vi "set_size.vi"(8 "error in (no error)":errorcluster, 9 "y":i32, 10 "x":i32, 11 "Image in":refnum<class "Image.lvclass">) -> (0 "error out":errorcluster, 3 "Image out":refnum<class "Image.lvclass">)   [LabVIEW 2010, in "Image.lvclass"]
uses:
  Image.lvclass
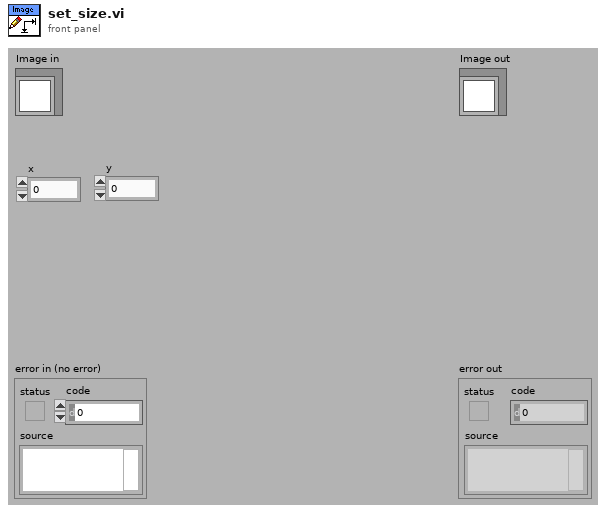
[diagram p1: front panel]
types:
  T1 = typedef "IMAQ Image.ctl" = refnum<image>
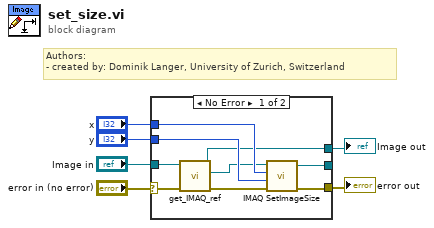
[diagram p0: block diagram]
diagram:
  # "Authors: \n- created by: Dominik Langer, University of Zurich, Switzerland"
  n1 = case shown="No Error" "error in (no error)" {
    selector: "error in (no error)" -> [w14 w17]
    tunnel: [w15 w17] -> w5
    tunnel: [w8 w16] -> w3
    tunnel: "Image in" -> [w12 w16]
    tunnel: "x" -> [w11 _]
    tunnel: "y" -> [w10 _]
    tunnel: [w7 _] -> _
    frame No Error {
      n2 = call-dynamic "get_IMAQ_ref.vi"("error in (no error)"=w14, "Image.lvclass in"=w12) -> ("error out"=w13:errorcluster, "Image"=w9:T1, "Image.lvclass out"=w8:refnum<class "Image.lvclass">)  [unwired: 7 out]
      n3 = call "IMAQ SetImageSize"("error in (no error)"=w13, "Y Resolution"=w10, "X Resolution"=w11, "Image"=w9) -> ("error out"=w15:errorcluster, "Image Out"=w7:T1)  [unwired: 1 out]
    }
    frame Error {
    }
  }
  "error out" <- w5
  "Image out" <- w3
